vi "StorageXMutationGetPath.vi"(1 "Node type":T1(ring)) -> (0 "appended path":path)   [LabVIEW 2017]
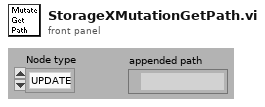
[diagram p1: front panel]
types:
  T1 = enum16{"UPDATE", "READ", "QUERY", "CREATE CHILD", "CREATE", "CONNECT", "DISCONNECT"}
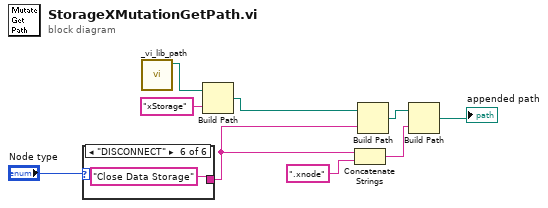
[diagram p0: block diagram]
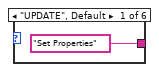
[diagram p2: hidden frame]
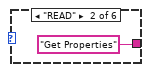
[diagram p3: hidden frame]
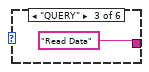
[diagram p4: hidden frame]
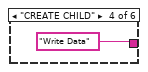
[diagram p5: hidden frame]
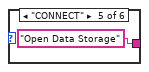
[diagram p6: hidden frame]
diagram:
  n1 = case shown="\"DISCONNECT\"" "Node type" {
    tunnel: ["Set Properties" ("name or relative path") "Get Properties" "Read Data" "Write Data" "Open Data Storage" "Close Data Storage"] -> w7
    frame "UPDATE", Default {
    }
    frame "READ" {
    }
    frame "QUERY" {
    }
    frame "CREATE CHILD" {
    }
    frame "CONNECT" {
    }
    frame "DISCONNECT" {
    }
  }
  n2 = call <vilib>:"_vi_lib_path.vi"() -> ("lvStorage.llb"=w4:path)  [unwired: 6 in, 1 out]
  n3 = Build Path(base path=w4, name or relative path="xStorage") -> (appended path=w2:path)
  n4 = Concatenate Strings(w7, ".xnode" ("string")) -> (w9:string)
  n5 = Build Path(base path=w2, name or relative path=w7) -> (appended path=w1:path)
  n6 = Build Path(base path=w1, name or relative path=w9) -> (appended path=→"appended path":path)
